vi "SiosIfmEnableEdlenCorrection.vi"(0 "On/Off":bool, 1 "Channel":i32(knob) scale=1.0..4.0, 2 "Device Number":i32) -> ()   [LabVIEW 2009]
uses:
  siosifm.dll
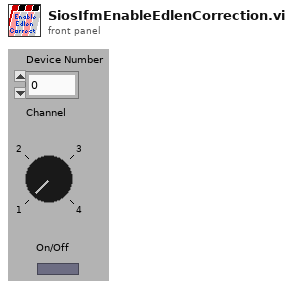
[diagram p1: front panel]
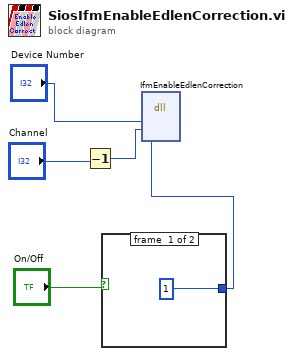
[diagram p0: block diagram]
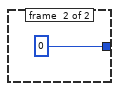
[diagram p2: hidden frame]
diagram:
  n1 = Decrement(x="Channel") -> (x-1=w3:i32)
  n2 = case shown="False" "On/Off" {
    tunnel: [1 0] -> w1
    frame #0 {
    }
    frame #1 {
    }
  }
  n3 = dll-call lib="C:/WORK/Artem/RE-10/SIOS_IfmDLL/siosifm.dll" fn="IfmEnableEdlenCorrection"("devNumber"="Device Number", "channel"=w3, "on"=w1) -> ()  [unwired: 7 in, 2 out]
